vi "graph.vi"() -> ()   [LabVIEW 2015]
panel:
  out "Waveform Chart":dbl(graph)
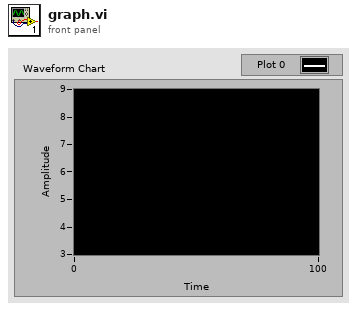
[diagram p1: front panel]
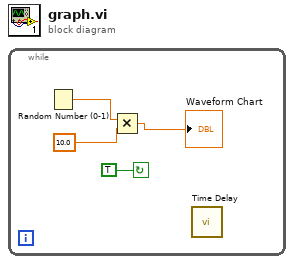
[diagram p0: block diagram]
diagram:
  n1 = while {
    stop <- TRUE continue-if-true
    n2 = Random Number (0-1)() -> (number: 0 to 1=w4:dbl)
    n3 = Multiply(x=w4, y=10.0 ("x*y")) -> (x*y=→"Waveform Chart":dbl)
    n4 = call "Time Delay"() -> ()  [unwired: 11 in, 1 out]
  }
